vi "BoardToPictures.vi"(8 "error in (no error)":errorcluster, 10 "Board":T1[][](array[typedef]), 11 "BoardDisplay in":refnum<class "BoardDisplay.lvclass">) -> (0 "error out":errorcluster, 2 "BoardVisulalization":picture[][](array[picture]), 3 "BoardDisplay out":refnum<class "BoardDisplay.lvclass">)   [LabVIEW 2015, in "TronviewPresentation.lvlib" / "BoardDisplay.lvclass"]
uses:
  BoardDisplay.lvclass
  TrajectoryBoardField.ctl
  TrajectoryFieldType.ctl
  TronVIEWBotAPI/MovementDirection.ctl
  BoardDisplay.lvclass/BoardDisplay.ctl
  TronVIEWBotAPI/TronVIEWBotAPI.lvlib
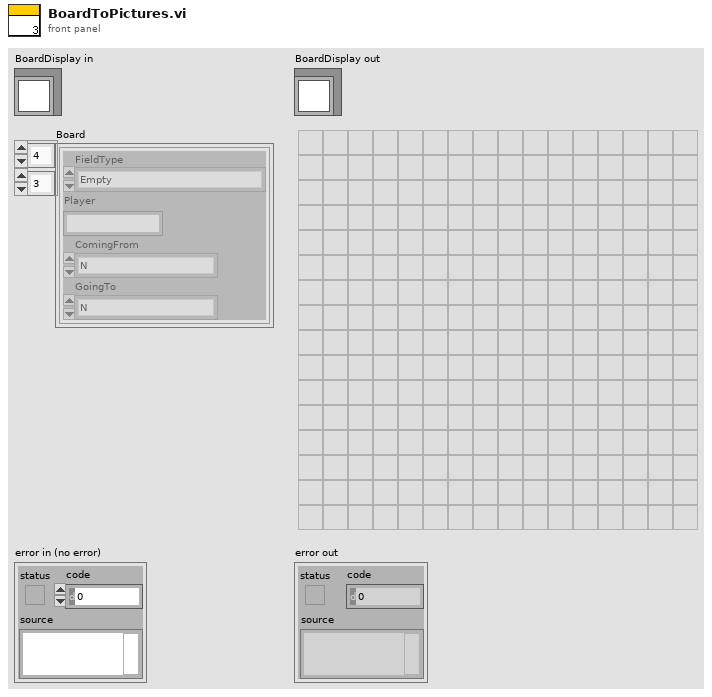
[diagram p1: front panel]
types:
  T1 = typedef "TronviewPresentation.lvlib/BoardDisplay.lvclass/TrajectoryBoardField.ctl" = cluster{"FieldType":T2, "Player":string, "ComingFrom":T3, "GoingTo":T3}
  T2 = typedef "TronviewPresentation.lvlib/BoardDisplay.lvclass/TrajectoryFieldType.ctl" = enum16{"Empty", "Initial", "PlayerWall", "PlayerPosition"}
  T3 = typedef "TronVIEWBotAPI.lvlib/MovementDirection.ctl" = enum16{"N", "S", "W", "E"}
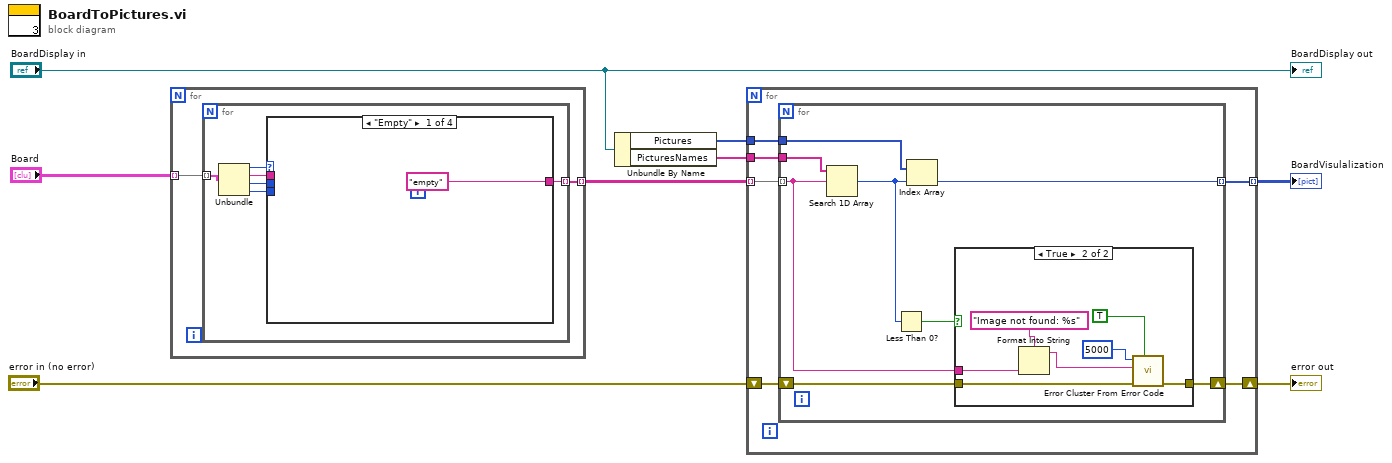
[diagram p0: block diagram]
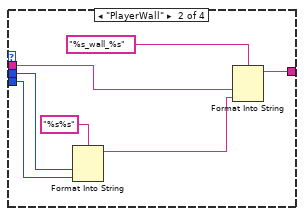
[diagram p2: hidden frame]
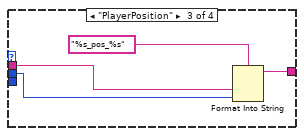
[diagram p3: hidden frame]
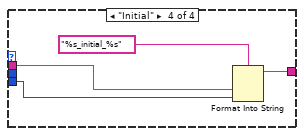
[diagram p4: hidden frame]
diagram:
  n1 = for {
    tunnel: [w10] -> w8 mode=indexing
    tunnel: "Board" -> [w9] mode=indexing
    n2 = for {
      tunnel: [w16] -> w10 mode=indexing
      tunnel: w9 -> [w14] mode=indexing
      n3 = Unbundle(w14) -> ("FieldType"=w13:T2, "Player"=w15:string, "ComingFrom"=w12:T3, "GoingTo"=w11:T3)
      n4 = case shown="\"Empty\"" w13 {
        tunnel: ["empty" w22 w26 w30] -> w16
        tunnel: w15 -> [_ w23 w27 w31]
        tunnel: w12 -> [_ w19 w25 _]
        tunnel: w11 -> [_ w20 _ w29]
        frame "Empty" {
        }
        frame "PlayerWall" {
          n5 = Format Into String(format string="%s%s", w19, w20) -> (resulting string=w18:string)  [unwired: 2 in, 1 out]
          n6 = Format Into String(format string="%s_wall_%s", w23, w18) -> (resulting string=w22:string)  [unwired: 2 in, 1 out]
        }
        frame "PlayerPosition" {
          n7 = Format Into String(format string="%s_pos_%s", w27, w25) -> (resulting string=w26:string)  [unwired: 2 in, 1 out]
        }
        frame "Initial" {
          n8 = Format Into String(format string="%s_initial_%s", w31, w29) -> (resulting string=w30:string)  [unwired: 2 in, 1 out]
        }
      }
    }
  }
  n9 = Unbundle By Name("BoardDisplay in") -> ("Pictures"=w4:picture[], "PicturesNames"=w5:string[])
  n10 = for {
    tunnel: w8 -> [w38] mode=indexing
    tunnel: w5 -> [w37]
    tunnel: w4 -> [w36]
    tunnel: [w35] -> w3 mode=indexing
    shift-right: [w34] -> w1
    shift-left: "error in (no error)" -> [w33]
    n11 = for {
      tunnel: w38 -> [w39] mode=indexing
      tunnel: w37 -> [w46]
      tunnel: w36 -> [w45]
      tunnel: [w44] -> w35 mode=indexing
      shift-right: [w41] -> w34
      shift-left: w33 -> [w43]
      n12 = Search 1D Array(1D array=w46, element=w39) -> (index of element=w42:i32)  [unwired: 1 in]
      n13 = Less Than 0?(x=w42) -> (x < 0?=w40:bool)
      n14 = Index Array(array=w45, index=w42) -> (element=w44:picture)
      n15 = case shown="True" w40 {
        tunnel: w43 -> [w47 w54]
        tunnel: [w47 w53] -> w41
        tunnel: w39 -> [_ w50]
        frame False {
        }
        frame True {
          n16 = Format Into String(format string="Image not found: %s" ("error message (\"\")"), w50) -> (resulting string=w49:string)  [unwired: 2 in, 1 out]
          n17 = call <vilib>:"Error Cluster From Error Code.vi"("show call chain? (False)"=TRUE, "error in (no error)"=w54, "error message (\"\")"=w49, "error code (0)"=5000) -> ("error out"=w53:errorcluster)  [unwired: 5 in]
        }
      }
    }
  }
  "error out" <- w1
  "BoardVisulalization" <- w3
  "BoardDisplay out" <- "BoardDisplay in"
